vi "CustomPathMath.vi"(0 "Total DataPoints":i32, 1 "Datapoint Index within Path":i32, 2 "Current Position":dbl, 3 "Input Position":dbl, 4 "A/D Rate":dbl) -> (14 "Calculated Position":dbl)   [LabVIEW 2012]
panel:
  # "Nano-Route™ 3D"
  # "Custom Path Generating SubVI"
  # "Standard Inputs"
  # "Required Output"
  # "Custom Inputs"
  # "Custom Outputs"
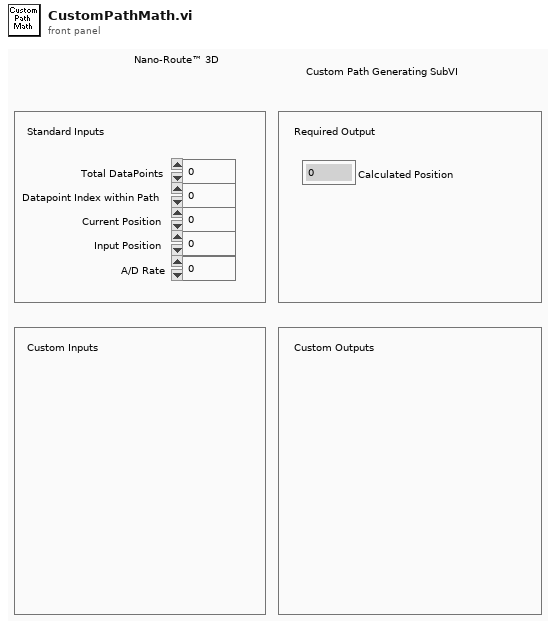
[diagram p1: front panel]
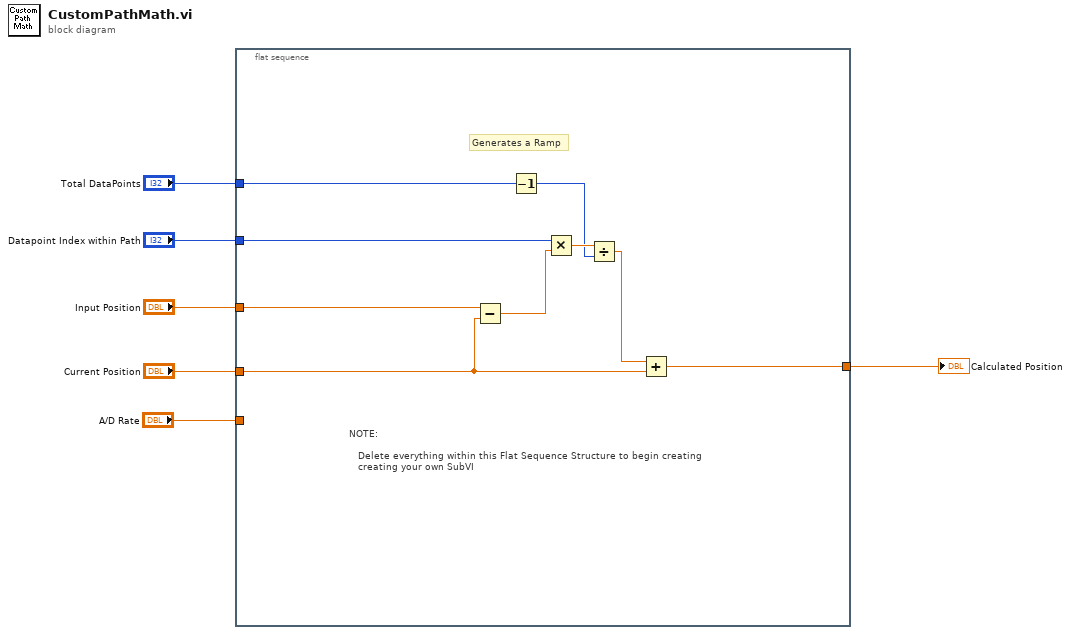
[diagram p0: block diagram]
diagram:
  n1 = flat-sequence {
    tunnel: "Input Position" -> [w15]
    tunnel: "Total DataPoints" -> [w14]
    tunnel: "Datapoint Index within Path" -> [w13]
    tunnel: "Current Position" -> [w10]
    tunnel: [w7] -> w2
    tunnel: "A/D Rate" -> [_]
    frame #0 {
      # "NOTE:\n\n   Delete everything within this Flat Sequence Structure to begin creating\n   creating your own SubVI"
      # "Generates a Ramp"
      n2 = Subtract(x=w15, y=w10) -> (x-y=w8:dbl)
      n3 = Decrement(x=w14) -> (x-1=w11:i32)
      n4 = Multiply(x=w13, y=w8) -> (x*y=w12:dbl)
      n5 = Divide(x=w12, y=w11) -> (x/y=w9:dbl)
      n6 = Add(x=w9, y=w10) -> (x+y=w7:dbl)
    }
  }
  "Calculated Position" <- w2
